vi "Dummy.vi"   [LabVIEW 2015]
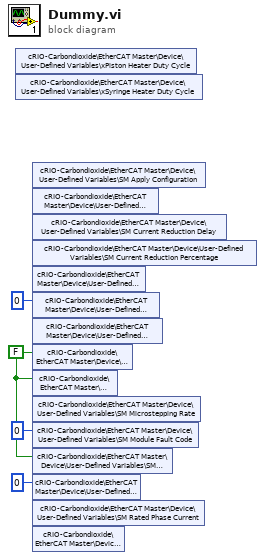
[diagram p0: block diagram]
diagram:
  w2 = FALSE ("xSM HOME")
  n1 = shared-variable "cRIO-Carbondioxide\\EtherCAT Master\\Device\\User-Defined Variables\\xPiston Heater Duty Cycle"() -> ()  [unwired: 1 in, 2 out]
  n2 = shared-variable "cRIO-Carbondioxide\\EtherCAT Master\\Device\\User-Defined Variables\\xSyringe Heater Duty Cycle"() -> ()  [unwired: 1 in, 2 out]
  n3 = shared-variable "cRIO-Carbondioxide\\EtherCAT Master\\Device\\User-Defined Variables\\SM Apply Configuration"() -> ()  [unwired: 1 in, 2 out]
  n4 = shared-variable "cRIO-Carbondioxide\\EtherCAT Master\\Device\\User-Defined Variables\\SM Clear Faults"() -> ()  [unwired: 1 in, 2 out]
  n5 = shared-variable "cRIO-Carbondioxide\\EtherCAT Master\\Device\\User-Defined Variables\\SM Current Reduction Delay"() -> ()  [unwired: 1 in, 2 out]
  n6 = shared-variable "cRIO-Carbondioxide\\EtherCAT Master\\Device\\User-Defined Variables\\SM Current Reduction Percentage"() -> ()  [unwired: 1 in, 2 out]
  n7 = shared-variable "cRIO-Carbondioxide\\EtherCAT Master\\Device\\User-Defined Variables\\SM Direction"() -> ()  [unwired: 1 in, 2 out]
  n8 = shared-variable "cRIO-Carbondioxide\\EtherCAT Master\\Device\\User-Defined Variables\\SM Drive Status"(u8 0 ("xSM Drive Status")) -> ()  [unwired: 1 in, 1 out]
  n9 = shared-variable "cRIO-Carbondioxide\\EtherCAT Master\\Device\\User-Defined Variables\\SM Enable Drive"() -> ()  [unwired: 1 in, 2 out]
  n10 = shared-variable "cRIO-Carbondioxide\\EtherCAT Master\\Device\\User-Defined Variables\\SM HOME"(w2) -> ()  [unwired: 1 in, 1 out]
  n11 = shared-variable "cRIO-Carbondioxide\\EtherCAT Master\\Device\\User-Defined Variables\\SM LIM"(w2) -> ()  [unwired: 1 in, 1 out]
  n12 = shared-variable "cRIO-Carbondioxide\\EtherCAT Master\\Device\\User-Defined Variables\\SM Microstepping Rate"() -> ()  [unwired: 1 in, 2 out]
  n13 = shared-variable "cRIO-Carbondioxide\\EtherCAT Master\\Device\\User-Defined Variables\\SM Module Fault Code"(u16 0 ("xSM Module Fault Code")) -> ()  [unwired: 1 in, 1 out]
  n14 = shared-variable "cRIO-Carbondioxide\\EtherCAT Master\\Device\\User-Defined Variables\\SM Module Fault?"(w2) -> ()  [unwired: 1 in, 1 out]
  n15 = shared-variable "cRIO-Carbondioxide\\EtherCAT Master\\Device\\User-Defined Variables\\SM Position"(0 ("xSM Position")) -> ()  [unwired: 1 in, 1 out]
  n16 = shared-variable "cRIO-Carbondioxide\\EtherCAT Master\\Device\\User-Defined Variables\\SM Rated Phase Current"() -> ()  [unwired: 1 in, 2 out]
  n17 = shared-variable "cRIO-Carbondioxide\\EtherCAT Master\\Device\\User-Defined Variables\\SM Ticks"() -> ()  [unwired: 1 in, 2 out]
